vi "FG_AnalysisSettgs.vi"(7 "Command":enum16{"Set", "Get", "Reset"}(ring), 8 "error in (no error)":errorcluster, 11 "Settings":T1) -> (0 "error out":errorcluster, 3 "Settings Out":T1)   [LabVIEW 2012]
uses:
  #TD_AnalysisSettings.ctl
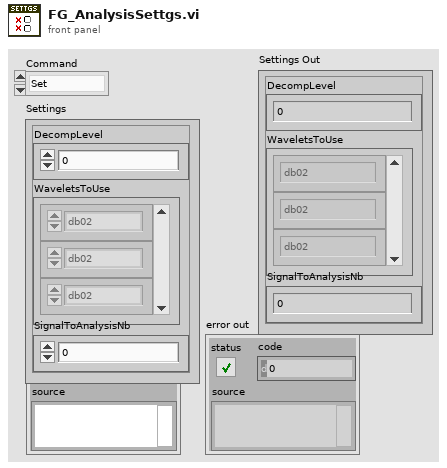
[diagram p1: front panel]
types:
  T1 = typedef "#TD_AnalysisSettings.ctl" = cluster{"DecompLevel":i32, "WaveletsToUse":enum16{"db02", "db03", "db04", "db05", "db06", "db07", "db08", "db09", "db10", "db11", "db12", "db13", "db14", "Haar", "bior1_3", "bior1_5", "bior2_2", "bior2_4", "bior2_6", "bior2_8", "bior3_1", "bior3_3", "bior3_5", "bior3_7", "bior3_9", "bior4_4 (FBI)", "bior5_5", "bior6_8", "coif1", "coif2", "coif3", "coif4", "coif5", "sym2", "sym3", "sym4", "sym5", "sym6", "sym7", "sym8"}[], "SignalToAnalysisNb":i32}
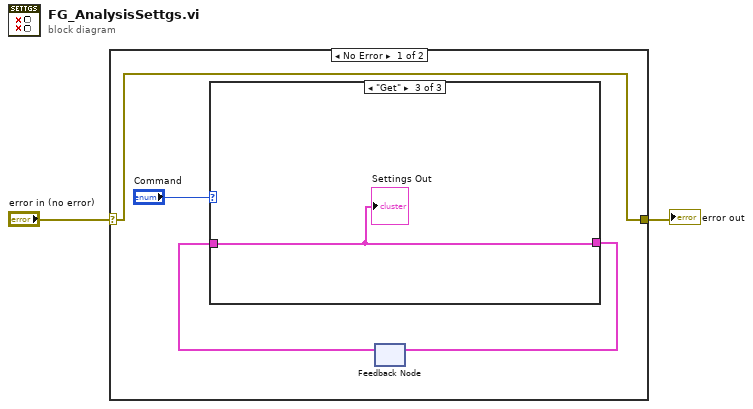
[diagram p0: block diagram]
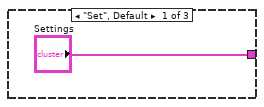
[diagram p2: hidden frame]
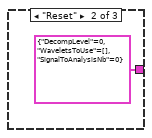
[diagram p3: hidden frame]
diagram:
  n1 = case shown="No Error" "error in (no error)" {
    selector: "error in (no error)" -> [w3 w10]
    tunnel: [w3 w10] -> w1
    frame No Error {
      n2 = feedback #1() -> (w4:T1)  [unwired: 1 in]
      n3 = case shown="\"Get\"" "Command" {
        tunnel: ["Settings" T1 {"DecompLevel"=0, "WaveletsToUse"=[], "SignalToAnalysisNb"=0} ("Settings") w9] -> w5
        tunnel: w4 -> [_ _ w9]
        frame "Set", Default {
        }
        frame "Reset" {
        }
        frame "Get" {
          "Settings Out" <- w9
        }
      }
      n4 = feedback-in #1(w5) -> ()
    }
    frame Error {
    }
  }
  "error out" <- w1
